vi "LIA Fgen Function Generator.vi"() -> ()   [LabVIEW 2017]
doc: "This example shows the Standard Function output mode. \n\nIt also shows some of the parameters which can be changed on the fly."
uses:
  <instrlib>/niFgen/niFgen.llb/niFgen Output Mode.ctl
panel:
  out "Output:Load Impedance 2":dbl
  out "Output:Load Impedance":dbl
  out "Output:Analog Path 2":i32(ring) items=["NIFGEN_VAL_MAIN_ANALOG_PATH", "NIFGEN_VAL_DIRECT_ANALOG_PATH", "NIFGEN_VAL_FIXED_LOW_GAIN_ANALOG_PATH", "NIFGEN_VAL_FIXED_HIGH_GAIN_ANALOG_PATH"]
  out "Output:Analog Path":i32(ring) items=["NIFGEN_VAL_MAIN_ANALOG_PATH", "NIFGEN_VAL_DIRECT_ANALOG_PATH", "NIFGEN_VAL_FIXED_LOW_GAIN_ANALOG_PATH", "NIFGEN_VAL_FIXED_HIGH_GAIN_ANALOG_PATH"]
  in  "Duty Cycle (%)":dbl(knob)=5.0 min=0.0 max=100.0 scale=0.0..100.0 scale format="%.1f"
  in  "FGEN Resource Name 2":refnum<k15>="Dev2" caption="FGEN Resource Name"
  in  "DC Offset (V) 2":dbl(knob) caption="DC Offset (V)" min=-6.0 max=6.0 scale=-6.0..6.0 scale format="%_1p"
  in  "Amplitude (Vp-p)  2":dbl(knob)=1.0 caption="Amplitude (Vp-p)" min=0.0 max=12.0 scale=0.0..12.0 scale format="%.1f"
  in  "Frequency (Hz) 2":dbl(knob)=100000.0 caption="Frequency (Hz)" min=9000.0 max=100000000.0 scale=0.0..100000000.0 scale format="%_1p"
  in  "Standard Waveform 2":u16(slide) caption="Standard Waveform" scale=0.0..6.0
  in  "Standard Waveform":u16(slide)=1 scale=0.0..6.0
  in  "Stop":bool
  in  "FGEN Resource Name":refnum<k15>="Dev1"
  in  "DC Offset (V)":dbl(knob) min=-6.0 max=6.0 scale=-6.0..6.0 scale format="%_1p"
  in  "Frequency (Hz)":dbl(knob)=100000.0 min=9000.0 max=100000000.0 scale=0.0..100000000.0 scale format="%_1p"
  in  "Amplitude (Vp-p)":dbl(knob)=1.0 min=0.0 max=12.0 scale=0.0..12.0 scale format="%.1f"
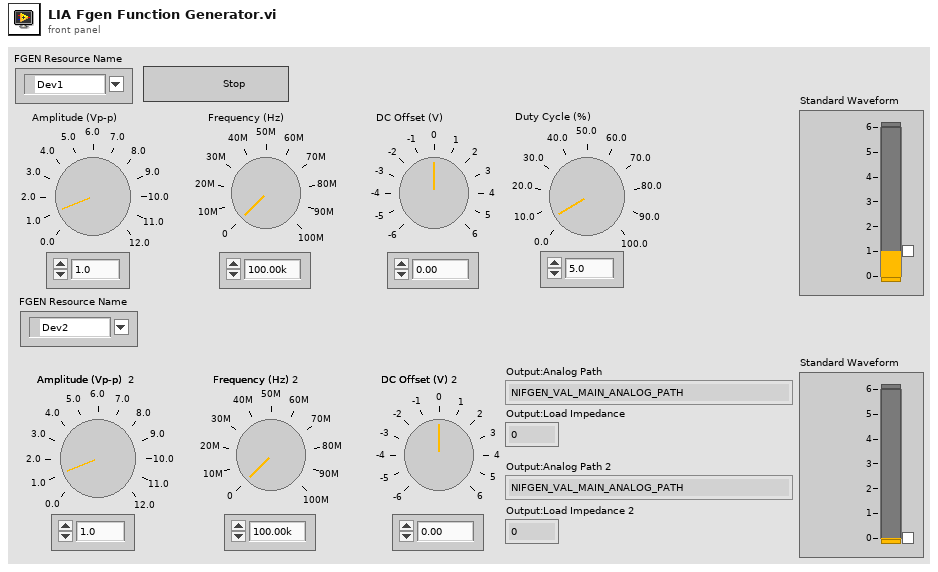
[diagram p1: front panel]
types:
  T1 = typedef "niFgen Output Mode.ctl" = u32
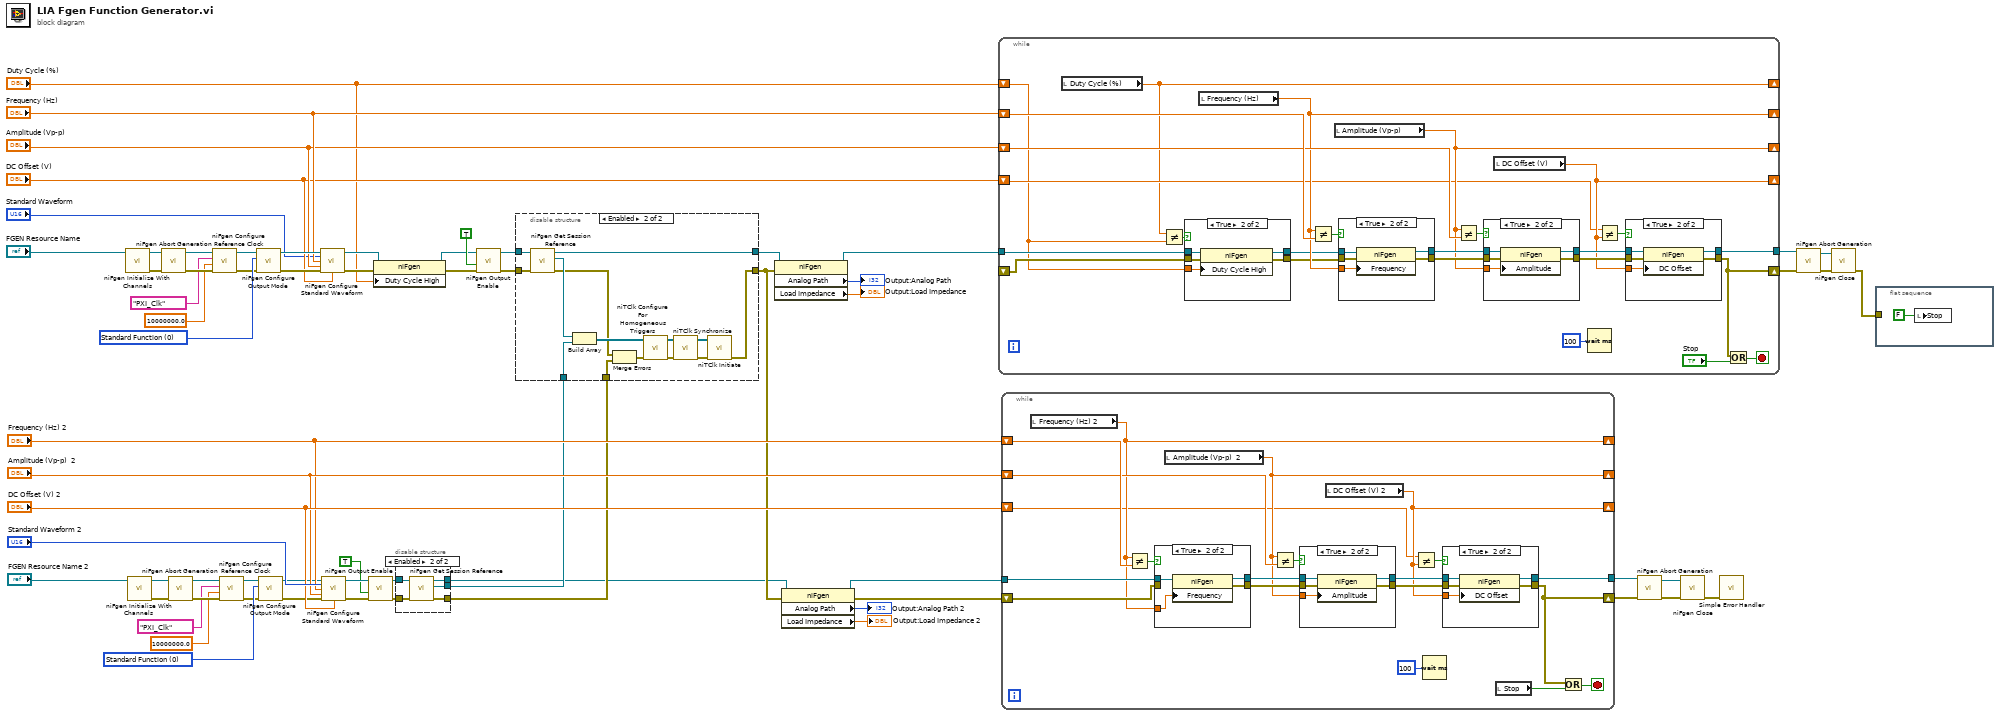
[diagram p0: block diagram]
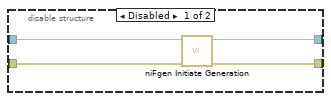
[diagram p2: hidden frame]
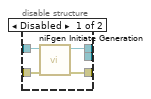
[diagram p3: hidden frame]
diagram:
  w38 = T1 0 items=["Standard Function", "Frequency List", "Arbitrary Waveform", "Arbitrary Sequence", "Script"] ("output mode")
  w59 = T1 0 items=["Standard Function", "Frequency List", "Arbitrary Waveform", "Arbitrary Sequence", "Script"] ("output mode")
  n1 = call <instrlib>:"niFgen Initialize With Channels.vi"("Resource Name"="FGEN Resource Name") -> ("error out"=w52:errorcluster, "Instrument Handle Out"=w51:refnum<k15>)  [unwired: 9 in]
  n2 = call <instrlib>:"niFgen Initialize With Channels.vi"("Resource Name"="FGEN Resource Name 2") -> ("error out"=w47:errorcluster, "Instrument Handle Out"=w48:refnum<k15>)  [unwired: 9 in]
  n3 = call <instrlib>:"niFgen Abort Generation.vi"("error in (no error)"=w52, "Instrument Handle"=w51) -> ("error out"=w61:errorcluster, "Instrument Handle Out"=w19:refnum<k15>)  [unwired: 8 in]
  n4 = call <instrlib>:"niFgen Abort Generation.vi"("error in (no error)"=w47, "Instrument Handle"=w48) -> ("error out"=w36:errorcluster, "Instrument Handle Out"=w15:refnum<k15>)  [unwired: 8 in]
  n5 = call <instrlib>:"niFgen Configure Reference Clock.vi"("error in (no error)"=w61, "Reference Clock Frequency"=10000000.0, "Source"="PXI_Clk", "Instrument Handle"=w19) -> ("error out"=w20:errorcluster, "Instrument Handle Out"=w18:refnum<k15>)  [unwired: 6 in]
  n6 = call <instrlib>:"niFgen Configure Reference Clock.vi"("error in (no error)"=w36, "Reference Clock Frequency"=10000000.0, "Source"="PXI_Clk", "Instrument Handle"=w15) -> ("error out"=w16:errorcluster, "Instrument Handle Out"=w14:refnum<k15>)  [unwired: 6 in]
  n7 = call <instrlib>:"niFgen Configure Output Mode.vi"("error in (no error)"=w20, "Output Mode (default: 0=Standard Function)"=w59, "Instrument Handle"=w18) -> ("error out"=w65:errorcluster, "Instrument Handle Out"=w63:refnum<k15>)  [unwired: 6 in]
  n8 = call <instrlib>:"niFgen Configure Output Mode.vi"("error in (no error)"=w16, "Output Mode (default: 0=Standard Function)"=w38, "Instrument Handle"=w14) -> ("error out"=w32:errorcluster, "Instrument Handle Out"=w34:refnum<k15>)  [unwired: 6 in]
  n9 = call <instrlib>:"niFgen Configure Standard Waveform.vi"("Instrument Handle"=w63, "Waveform"="Standard Waveform", "Frequency"="Frequency (Hz)", "Amplitude"="Amplitude (Vp-p)", "error in (no error)"=w65, "DC Offset"="DC Offset (V)") -> ("Instrument Handle Out"=w28:refnum<k15>, "error out"=w26:errorcluster)  [unwired: 8 in]
  n10 = call <instrlib>:"niFgen Configure Standard Waveform.vi"("Instrument Handle"=w34, "Waveform"="Standard Waveform 2", "Frequency"="Frequency (Hz) 2", "Amplitude"="Amplitude (Vp-p)  2", "error in (no error)"=w32, "DC Offset"="DC Offset (V) 2") -> ("Instrument Handle Out"=w40:refnum<k15>, "error out"=w39:errorcluster)  [unwired: 8 in]
  n11 = call <instrlib>:"niFgen Output Enable.vi"("error in (no error)"=w39, "Output Enable (default: True)"=TRUE ("output enable"), "Instrument Handle"=w40) -> ("error out"=w33:errorcluster, "Instrument Handle Out"=w35:refnum<k15>)  [unwired: 7 in]
  n12 = property class="niFgen"(reference=w28, error in=w26, "Duty Cycle High"="Duty Cycle (%)") -> (reference out=w27:refnum<k15>, error out=w25:errorcluster)
  n13 = disable-structure shown="Enabled" {
    disable-tunnel: [w71 w73] -> w22
    disable-tunnel: [w70 w75] -> w5
    disable-tunnel: w35 -> [w69 w76]
    disable-tunnel: w33 -> [w68 w74]
    disable-tunnel: [_ w72] -> w23
    frame Disabled {
      n14 = call <instrlib>:"niFgen Initiate Generation.vi"("error in (no error)"=w68, "Instrument Handle"=w69) -> ("error out"=w71:errorcluster, "Instrument Handle Out"=w70:refnum<k15>)  [unwired: 8 in]
    }
    frame Enabled {
      n15 = call <instrlib>:"niFgen Get Session Reference.vi"("error in (no error)"=w74, "Instrument Handle"=w76) -> ("error out"=w73:errorcluster, "Session Reference"=w72:refnum<k20>, "Instrument Handle Out"=w75:refnum<k15>)  [unwired: 7 in]
    }
  }
  n16 = call <instrlib>:"niFgen Output Enable.vi"("error in (no error)"=w25, "Output Enable (default: True)"=TRUE ("output enable"), "Instrument Handle"=w27) -> ("error out"=w64:errorcluster, "Instrument Handle Out"=w62:refnum<k15>)  [unwired: 7 in]
  n17 = disable-structure shown="Enabled" {
    disable-tunnel: w64 -> [w80 w91]
    disable-tunnel: w62 -> [w79 w92]
    disable-tunnel: [w78 w90] -> w10
    disable-tunnel: [w77 w81] -> w6
    disable-tunnel: w23 -> [_ w87]
    disable-tunnel: w22 -> [_ w82]
    frame Disabled {
      n18 = call <instrlib>:"niFgen Initiate Generation.vi"("error in (no error)"=w80, "Instrument Handle"=w79) -> ("error out"=w77:errorcluster, "Instrument Handle Out"=w78:refnum<k15>)  [unwired: 8 in]
    }
    frame Enabled {
      n19 = call <instrlib>:"niFgen Get Session Reference.vi"("error in (no error)"=w91, "Instrument Handle"=w92) -> ("error out"=w83:errorcluster, "Session Reference"=w84:refnum<k20>, "Instrument Handle Out"=w90:refnum<k15>)  [unwired: 7 in]
      n20 = Build Array(w84, w87) -> (w86:refnum<k20>[])
      n21 = Merge Errors(w83, w82) -> (w85:errorcluster)
      n22 = call <instrlib>:"niTClk Configure For Homogeneous Triggers.vi"("error in (no error)"=w85, "sessions"=w86) -> ("error out"=w93:errorcluster, "sessions out"=w89:refnum<k20>[])  [unwired: 8 in]
      n23 = call <instrlib>:"niTClk Synchronize.vi"("error in (no error)"=w93, "sessions"=w89) -> ("error out"=w94:errorcluster, "sessions out"=w88:refnum<k20>[])  [unwired: 8 in]
      n24 = call <instrlib>:"niTClk Initiate.vi"("error in (no error)"=w94, "sessions"=w88) -> ("error out"=w81:errorcluster)  [unwired: 8 in, 1 out]
    }
  }
  n25 = property class="niFgen"(reference=w10, error in=w6) -> (reference out=w9:refnum<k15>, "Analog Path"=→"Output:Analog Path":i32, "Load Impedance"=→"Output:Load Impedance":dbl)  [unwired: 1 out]
  n26 = property class="niFgen"(reference=w5, error in=w6) -> (reference out=w4:refnum<k15>, error out=w3:errorcluster, "Analog Path"=→"Output:Analog Path 2":i32, "Load Impedance"=→"Output:Load Impedance 2":dbl)
  n27 = while {
    tunnel: w9 -> [w99]
    tunnel: [w115] -> w58
    shift-right: [w104] -> _
    shift-left: "Frequency (Hz)" -> [w113]
    shift-right: [w103] -> _
    shift-left: "Amplitude (Vp-p)" -> [w112]
    shift-right: [w102] -> _
    shift-left: "DC Offset (V)" -> [w101]
    shift-right: [w105] -> w55
    shift-left: _ -> [w114]
    shift-right: [w95] -> _
    shift-left: "Duty Cycle (%)" -> [w96]
    stop <- w106 stop-if-true
    n28 = local read "Duty Cycle (%)"() -> (w95:dbl)
    n29 = Not Equal?(x=w95, y=w96) -> (x != y?=w97:bool)
    n30 = case shown="True" w97 {
      tunnel: w114 -> [w120 w126]
      tunnel: [w120 w125] -> w100
      tunnel: w99 -> [w121 w124]
      tunnel: [w121 w123] -> w98
      tunnel: w96 -> [_ w122]
      frame False {
      }
      frame True {
        n31 = property class="niFgen"(reference=w124, error in=w126, "Duty Cycle High"=w122) -> (reference out=w123:refnum<k15>, error out=w125:errorcluster)
      }
    }
    n32 = local read "Frequency (Hz)"() -> (w104:dbl)
    n33 = Not Equal?(x=w104, y=w113) -> (x != y?=w111:bool)
    n34 = local read "Amplitude (Vp-p)"() -> (w103:dbl)
    n35 = case shown="True" w111 {
      tunnel: [w142 w147] -> w116
      tunnel: [w141 w146] -> w117
      tunnel: w98 -> [w142 w145]
      tunnel: w100 -> [w141 w143]
      tunnel: w104 -> [_ w144]
      frame False {
      }
      frame True {
        n36 = property class="niFgen"(reference=w145, error in=w143, "Frequency"=w144) -> (reference out=w147:refnum<k15>, error out=w146:errorcluster)
      }
    }
    n37 = Not Equal?(x=w103, y=w112) -> (x != y?=w110:bool)
    n38 = case shown="True" w110 {
      tunnel: w116 -> [w135 w140]
      tunnel: w117 -> [w134 w139]
      tunnel: [w134 w138] -> w118
      tunnel: [w135 w137] -> w119
      tunnel: w103 -> [_ w136]
      frame False {
      }
      frame True {
        n39 = property class="niFgen"(reference=w140, error in=w139, "Amplitude"=w136) -> (reference out=w137:refnum<k15>, error out=w138:errorcluster)
      }
    }
    n40 = local read "DC Offset (V)"() -> (w102:dbl)
    n41 = Wait (ms)(milliseconds to wait=u32 100) -> ()  [unwired: 1 out]
    n42 = Not Equal?(x=w101, y=w102) -> (x != y?=w109:bool)
    n43 = case shown="True" w109 {
      tunnel: w118 -> [w127 w133]
      tunnel: w119 -> [w128 w132]
      tunnel: [w128 w131] -> w115
      tunnel: [w127 w130] -> w105
      tunnel: w102 -> [_ w129]
      frame False {
      }
      frame True {
        n44 = property class="niFgen"(reference=w132, error in=w133, "DC Offset"=w129) -> (reference out=w131:refnum<k15>, error out=w130:errorcluster)
      }
    }
    n45 = Or(x=w105, y="Stop") -> (x .or. y?=w106:bool)
  }
  n46 = while {
    tunnel: w4 -> [w162]
    tunnel: [w163] -> w41
    shift-right: [w152] -> _
    shift-left: "Frequency (Hz) 2" -> [w160]
    shift-right: [w151] -> _
    shift-left: "Amplitude (Vp-p)  2" -> [w159]
    shift-right: [w150] -> _
    shift-left: "DC Offset (V) 2" -> [w149]
    shift-right: [w153] -> w44
    shift-left: w3 -> [w161]
    stop <- w154 stop-if-true
    n47 = local read "Frequency (Hz) 2"() -> (w152:dbl)
    n48 = Not Equal?(x=w152, y=w160) -> (x != y?=w158:bool)
    n49 = case shown="True" w158 {
      tunnel: [w183 w187] -> w164
      tunnel: [w182 w186] -> w165
      tunnel: w162 -> [w183 w185]
      tunnel: w161 -> [w182 _]
      tunnel: w152 -> [_ w184]
      frame False {
      }
      frame True {
        n50 = property class="niFgen"(reference=w185, "Frequency"=w184) -> (reference out=w187:refnum<k15>, error out=w186:errorcluster)  [unwired: 1 in]
      }
    }
    n51 = local read "Amplitude (Vp-p)  2"() -> (w151:dbl)
    n52 = Not Equal?(x=w151, y=w159) -> (x != y?=w157:bool)
    n53 = case shown="True" w157 {
      tunnel: w164 -> [w176 w181]
      tunnel: w165 -> [w175 w180]
      tunnel: [w175 w179] -> w166
      tunnel: [w176 w178] -> w167
      tunnel: w151 -> [_ w177]
      frame False {
      }
      frame True {
        n54 = property class="niFgen"(reference=w181, error in=w180, "Amplitude"=w177) -> (reference out=w178:refnum<k15>, error out=w179:errorcluster)
      }
    }
    n55 = local read "DC Offset (V) 2"() -> (w150:dbl)
    n56 = Not Equal?(x=w149, y=w150) -> (x != y?=w156:bool)
    n57 = Wait (ms)(milliseconds to wait=u32 100) -> ()  [unwired: 1 out]
    n58 = case shown="True" w156 {
      tunnel: w166 -> [w168 w174]
      tunnel: w167 -> [w169 w173]
      tunnel: [w169 w172] -> w163
      tunnel: [w168 w171] -> w153
      tunnel: w150 -> [_ w170]
      frame False {
      }
      frame True {
        n59 = property class="niFgen"(reference=w173, error in=w174, "DC Offset"=w170) -> (reference out=w172:refnum<k15>, error out=w171:errorcluster)
      }
    }
    n60 = local read "Stop"() -> (w148:bool)
    n61 = Or(x=w153, y=w148) -> (x .or. y?=w154:bool)
  }
  n62 = call <instrlib>:"niFgen Abort Generation.vi"("error in (no error)"=w44, "Instrument Handle"=w41) -> ("error out"=w30:errorcluster, "Instrument Handle Out"=w29:refnum<k15>)  [unwired: 8 in]
  n63 = call <instrlib>:"niFgen Close.vi"("error in (no error)"=w30, "Instrument Handle"=w29) -> ("error out"=w31:errorcluster)  [unwired: 9 in]
  n64 = call <vilib>:"Simple Error Handler.vi"("error in (no error)"=w31) -> ()  [unwired: 4 in, 5 out]
  n65 = call <instrlib>:"niFgen Abort Generation.vi"("error in (no error)"=w55, "Instrument Handle"=w58) -> ("error out"=w66:errorcluster, "Instrument Handle Out"=w67:refnum<k15>)  [unwired: 8 in]
  n66 = call <instrlib>:"niFgen Close.vi"("error in (no error)"=w66, "Instrument Handle"=w67) -> ("error out"=w21:errorcluster)  [unwired: 9 in]
  n67 = flat-sequence {
    tunnel: w21 -> [_]
    frame #0 {
      n68 = local write "Stop"(FALSE) -> ()
    }
  }
